vi "Main(Analysis_Debug2_Mode).vi"() -> ()   [LabVIEW 2015]
uses:
  Sub VI/buffer_mode.ctl
  <vilib>/Analysis/baseanly.llb/Mean (DBL).vi
  <vilib>/Utility/NIReport.llb/Append Text Table to Report (wrap).vi
  <vilib>/Utility/NIReport.llb/NI_report.lvclass
  <vilib>/Analysis/NI_AALBase.lvlib
panel:
  in  "Data Range Clear":bool
  in  "Auto Range":bool
  out "Range(min)":dbl caption="End - Start Time (min)"
  in  "Cursor Mode":enum16{"Free", "Sample"}(ring)
  out "Save as Task Time(sec)":dbl
  in  "Use Filter data":bool
  in  "Data Range Subset":bool
  in  "Range":dbl caption="Sample Range"
  in  "Analysis List":i32(listbox)
  in  "Data Range Addition":bool
  in  "Over-write":bool
  in  "Number of Data Down-Sampling":i32
  in  "Save As":bool
  in  "Refresh":bool
  in  "Delete":bool
  in  "Plot Display mode":T1(ring)
  in  "File Name":string(combo)
  in  "Analysis mode":u16(ring) items=["Sensor Response Linearity", "Sensor Hysteresis with No Dwell Time", "Sensor Hysteresis with Varying Dwell Time", "Reated Loading", "Drift with Set Temperature and Voltage", "Variation Due to Self-Heating", "Variation with Changing Voltage", "Electrical Noise"]
  in  "Start Analysis":bool
  in  "File Path":path
  out "XY 그래프":cluster{"Time(s)":dbl[], "calculation":u32[]}[](graph)
  # "V1.0"
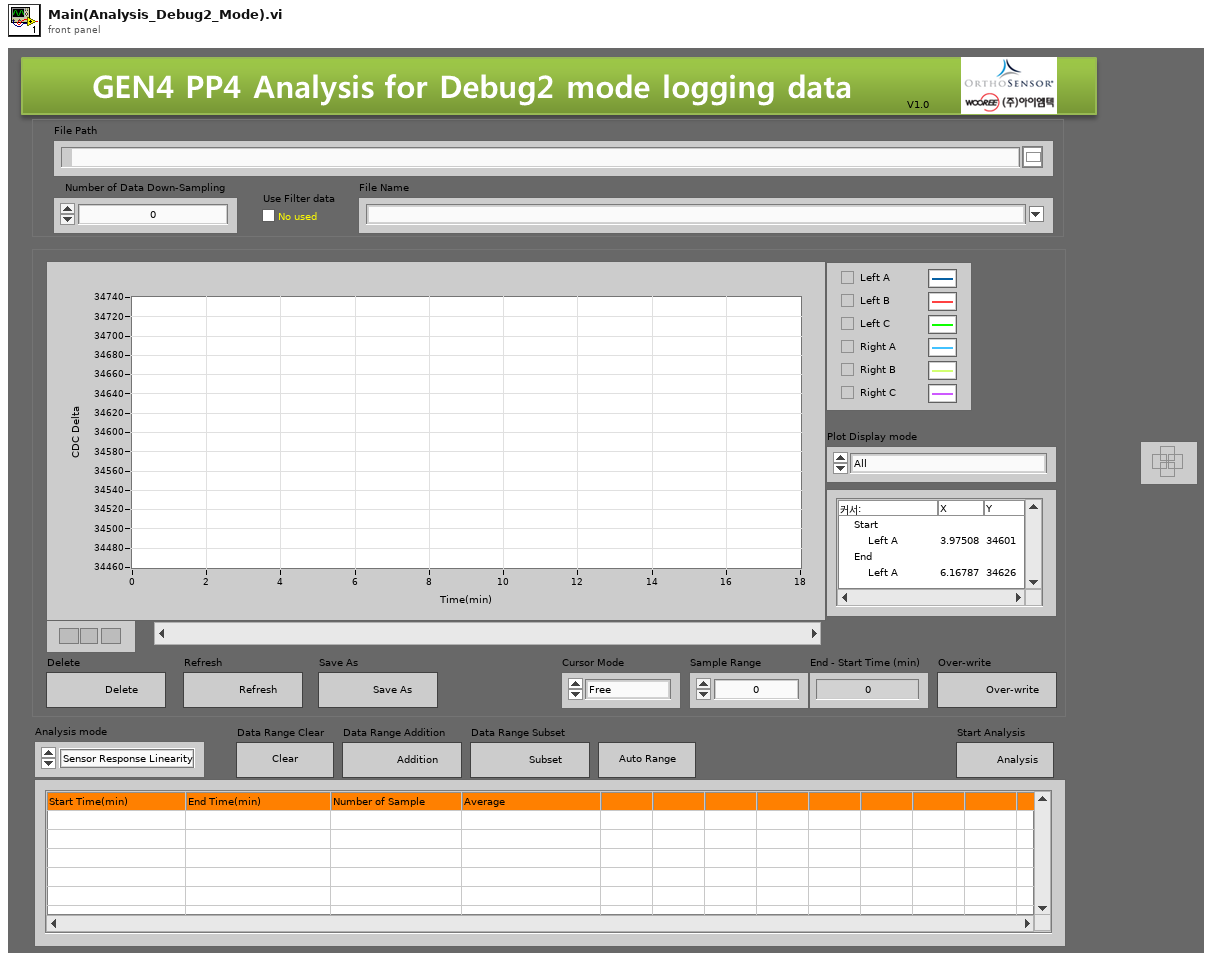
[diagram p1: front panel]
types:
  T1 = enum16{"All", "Left A", "Left B", "Left C", "Right A", "Right B", "Right C"}
  T2 = enum8{"Enabled", "Disabled", "Disabled and Grayed Out"}
  T3 = typedef "LVCursorListTypeDef.ctl" = cluster{"Name":string, "Color":u32, "Style":u8, "Point Style":u8, "Name Visible":bool, "Allow Drag":bool, "Cursor Mode":u32, "Plot":i32, "Index":i32, "Position":cluster{"X":dbl, "Y":dbl}, "X Scale":u32, "Y Scale":u32, "Watch Plots":i32[], "Watch All Plots":bool, "Plot Area":i32, "Label Offset":cluster{"X":dbl, "Y":dbl}}[]
  T4 = cluster{"Name":string, "Color":u32, "Style":u8, "Point Style":u8, "Name Visible":bool, "Allow Drag":bool, "Cursor Mode":u32, "Plot":i32, "Index":i32, "Position":cluster{"X":dbl, "Y":dbl}, "X Scale":u32, "Y Scale":u32, "Watch Plots":i32[], "Watch All Plots":bool, "Plot Area":i32, "Label Offset":cluster{"X":dbl, "Y":dbl}}
  T5 = typedef "buffer_mode.ctl" = enum16{"Clear", "Init", "Add 2nd data", "Delete", "Output"}
  T6 = cluster{"position (excel)":cluster{"row":i32, "column":i32}, "name (excel)":string, "bookmark (word)":string}
  T7 = enum16{"maximized", "minimized", "normal", "no change"}
  T8 = enum16{"Standard Report", "HTML", "Word", "Excel"}
  T9 = cluster{"Name":string, "Color":u32, "Style":u8, "Point Style":u8, "Name Visible":bool, "Allow Drag":bool, "Cursor Mode":u32, "Plot":i32, "Index":i32, "Position":cluster{"X":dbl, "Y":dbl}, "X Scale":u32, "Y Scale":u32, "Watch Plots":i32[], "Watch All Plots":bool, "Plot Area":i32, "Label Offset":cluster{"X":dbl, "Y":dbl}}[]
  T10 = cluster{"Timeline out":dbl[], "Counts out":u32[]}
  T11 = cluster{"Timeline out":dbl[], "Counts out":u32[]}[]
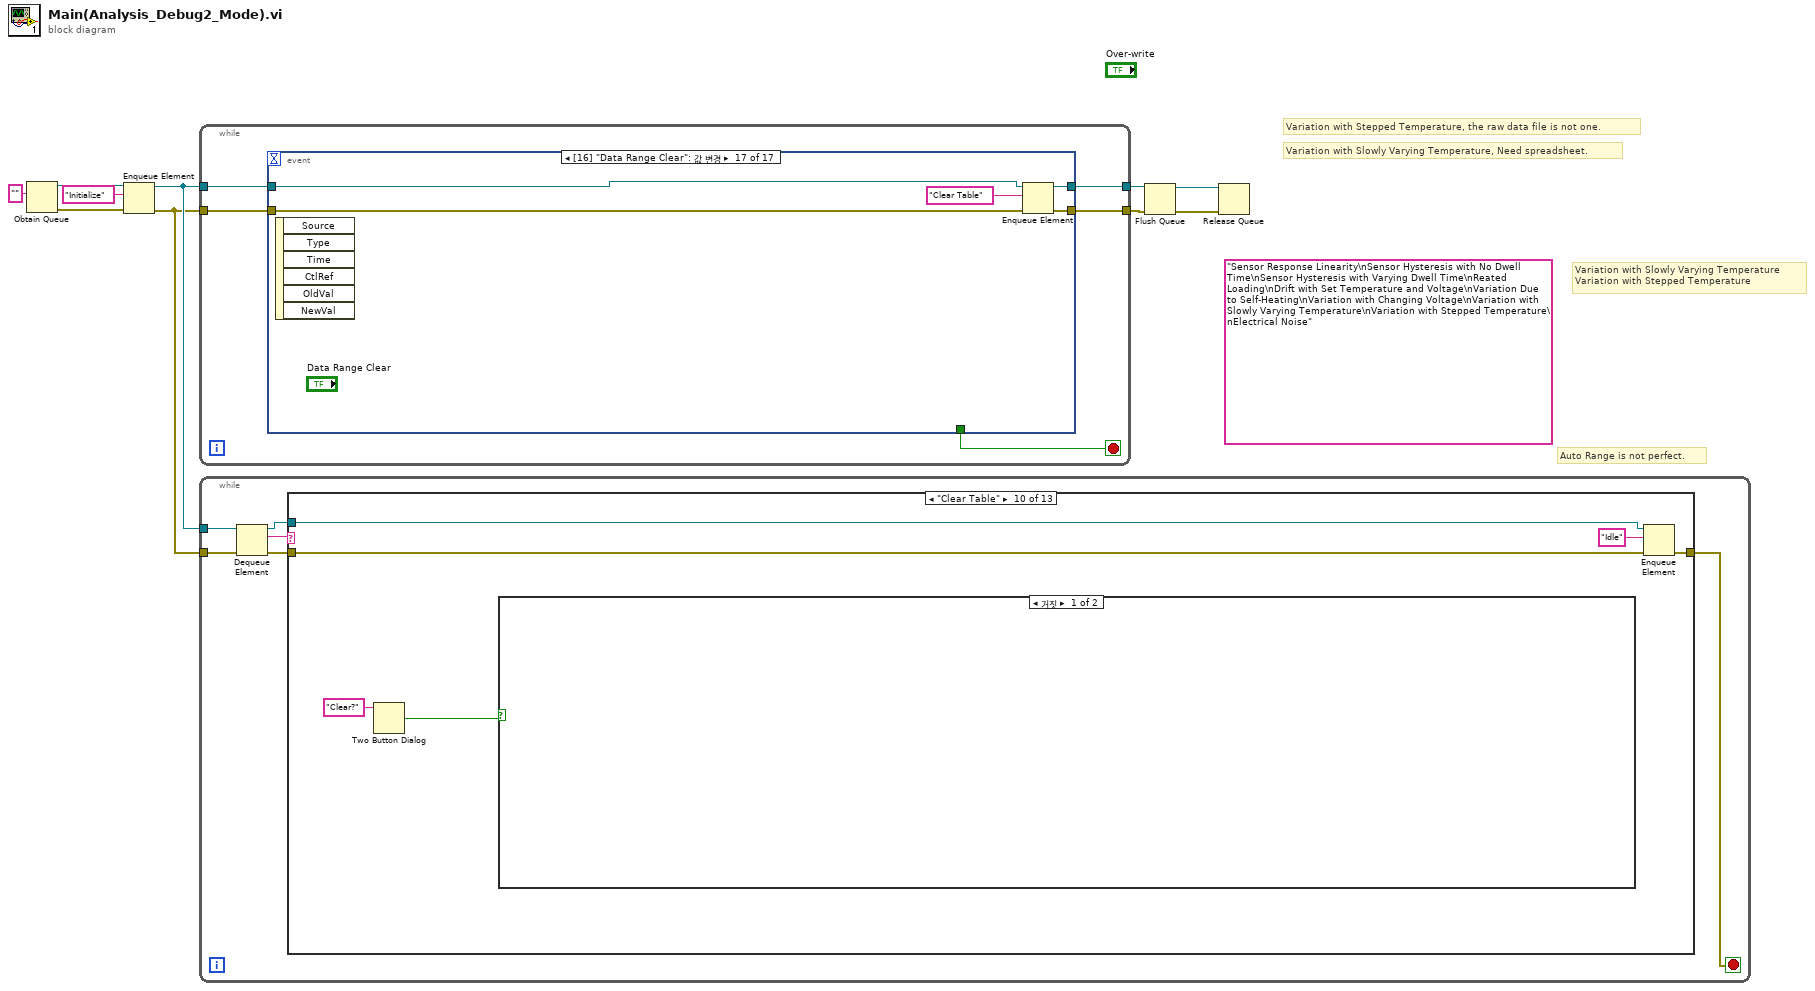
[diagram p0: block diagram]
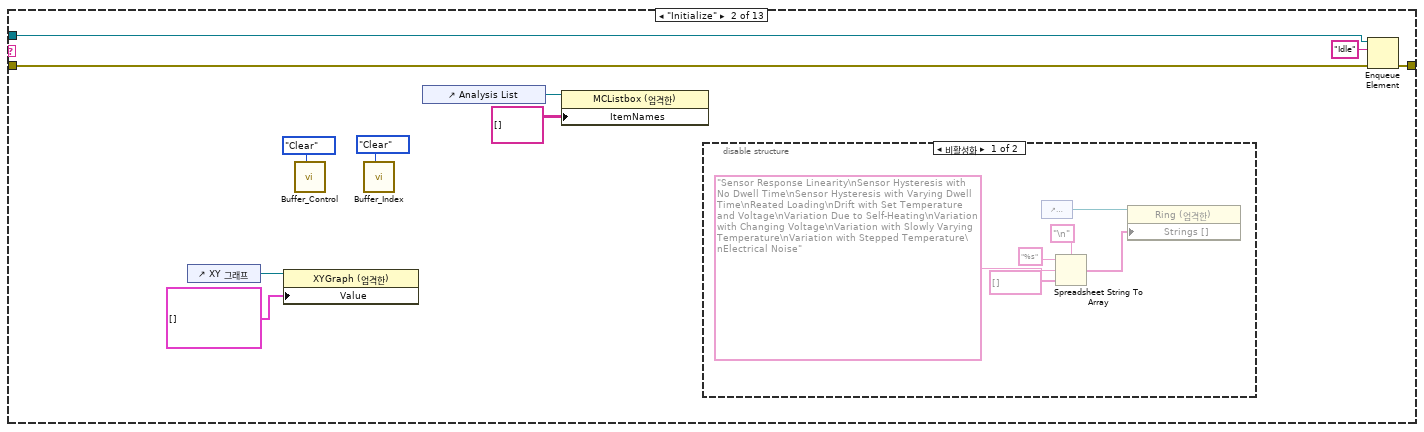
[diagram p3: hidden frame]
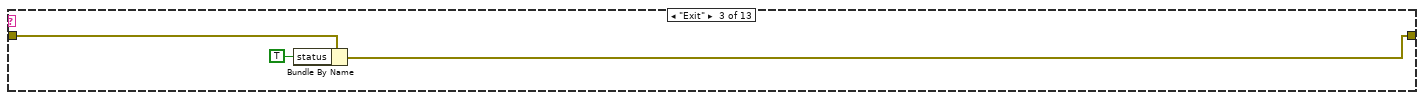
[diagram p5: hidden frame]
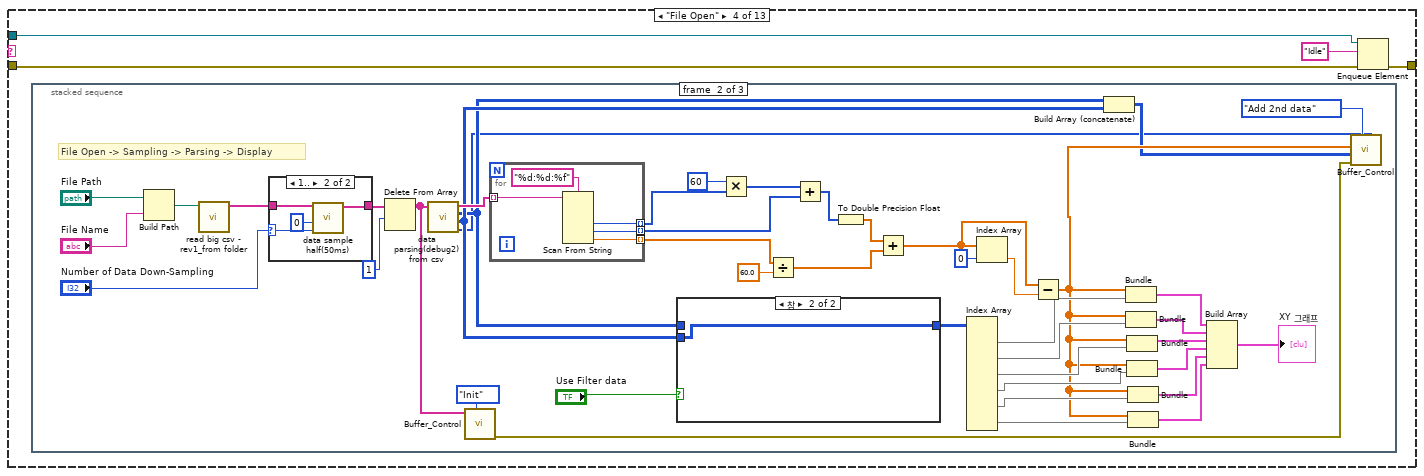
[diagram p6: hidden frame]
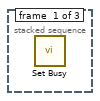
[diagram p7: hidden frame]
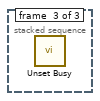
[diagram p10: hidden frame]
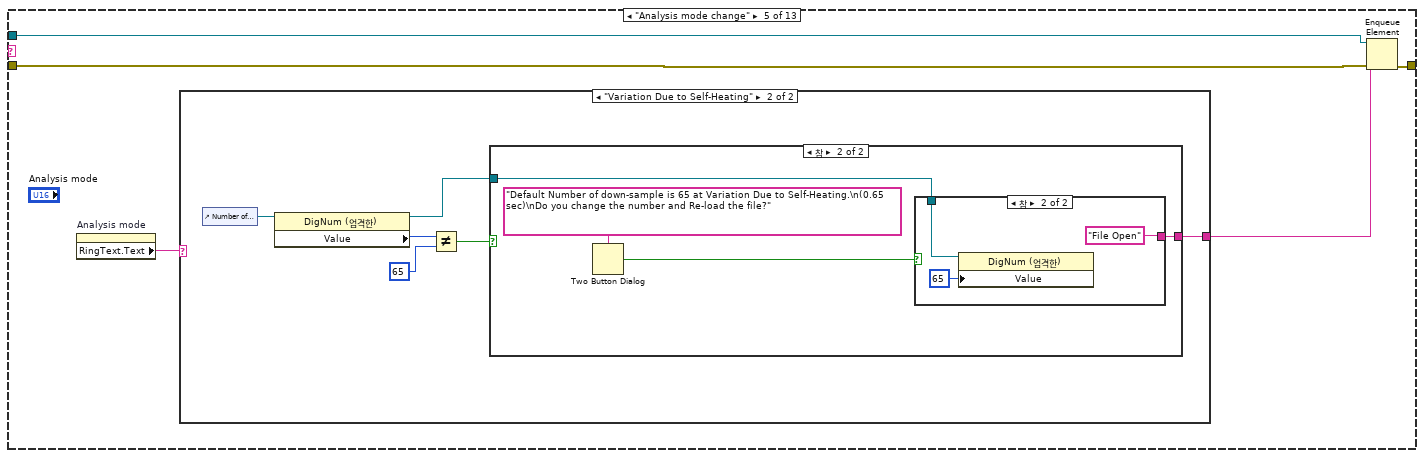
[diagram p11: hidden frame]
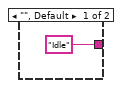
[diagram p12: hidden frame]
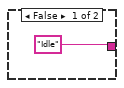
[diagram p13: hidden frame]
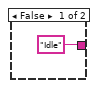
[diagram p14: hidden frame]
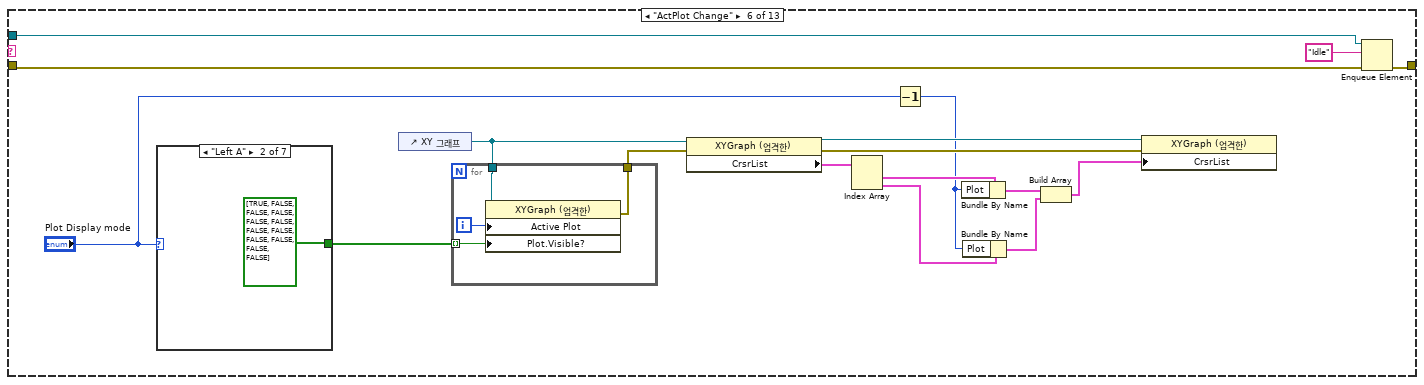
[diagram p15: hidden frame]
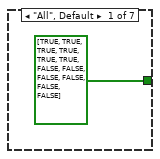
[diagram p16: hidden frame]
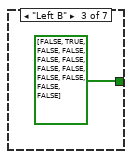
[diagram p17: hidden frame]
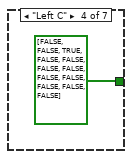
[diagram p18: hidden frame]
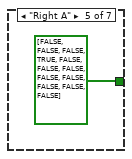
[diagram p19: hidden frame]
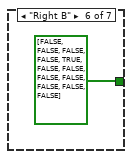
[diagram p20: hidden frame]
diagram:
  (unwired) "Sensor Response Linearity\nSensor Hysteresis with No Dwell Time\nSensor Hysteresis with Varying Dwell Time\nReated Loading\nDrift with Set Temperature and Voltage\nVariation Due to Self-Heating\nVariation with Changing Voltage\nVariation with Slowly Varying Temperature\nVariation with Stepped Temperature\nElectrical Noise" ("스프레드시트 문자열")
  # "Variation with Slowly Varying Temperature, Need spreadsheet."
  # "Variation with Stepped Temperature, the raw data file is not one."
  # "Variation with Slowly Varying Temperature\nVariation with Stepped Temperature"
  # "Auto Range is not perfect."
  n1 = Obtain Queue(element data type="" ("element")) -> (queue out=w10:refnum<queue>, error out=w9:errorcluster)  [unwired: 4 in, 1 out]
  n2 = Enqueue Element(queue=w10, element="Initialize", error in (no error)=w9) -> (queue out=w2:refnum<queue>, error out=w1:errorcluster)  [unwired: 1 in, 1 out]
  n3 = while {
    tunnel: w2 -> [w15]
    tunnel: [w14] -> w4
    tunnel: w1 -> [w13]
    tunnel: [w12] -> w3
    stop <- w11 stop-if-true
    n4 = event shown="[16] \"Data Range Clear\": 값 변경" {
      selector: _ -> [_ _ _ _ _ _ _ _ _ _ _ _ _ _ _ _ _]
      dyn-events: _ -> [_ _ _ _ _ _ _ _ _ _ _ _ _ _ _ _ _]
      timeout: _ -> [_ _ _ _ _ _ _ _ _ _ _ _ _ _ _ _ _]
      tunnel: w15 -> [w17 w18 w26 w31 w39 w51 w67 w72 w77 w85 w94 w98 w108 w112 w119 w124 w130]
      tunnel: [w17 w20 w28 w33 w38 w52 w68 w73 w78 w88 w95 w101 w109 w114 w122 w126 w131] -> w14
      tunnel: w13 -> [w16 w19 w27 w32 w40 w50 w66 w71 w76 w86 w93 w99 w107 w113 w120 w125 w129]
      tunnel: [w16 w21 w29 w34 w41 w53 w69 w74 w79 w87 w96 w100 w110 w115 w121 w127 w132] -> w12
      tunnel: [_ TRUE _ _ _ _ _ _ _ _ _ _ _ _ _ _ _] -> w11
      event Timeout {
        n5 = event-data() -> ()  [unwired: 1 in, 3 out]
      }
      event Panel Close {
        n6 = event-data() -> ()  [unwired: 1 in, 4 out]
        n7 = Enqueue Element(queue=w18, element="Exit", error in (no error)=w19) -> (queue out=w20:refnum<queue>, error out=w21:errorcluster)  [unwired: 1 in, 1 out]
      }
      event "File Name": Value Change {
        # "File Open -> Sampling -> Parsing -> Display"
        n8 = event-data() -> ()  [unwired: 1 in, 1 out]
        n9 = control-ref of="XY 그래프"() -> (w25:refnum<vi>)
        n10 = property class="XYGraph (엄격한)"(reference=w25, "Value"=cluster{"Time(s)":dbl[], "calculation":u32[]}[] [] ("값")) -> ()  [unwired: 1 in, 2 out]
        n11 = Enqueue Element(queue=w26, element="File Open", error in (no error)=w27) -> (queue out=w28:refnum<queue>, error out=w29:errorcluster)  [unwired: 1 in, 1 out]
      }
      event "Delete": Value Change {
        n12 = event-data() -> ()  [unwired: 1 in, 6 out]
        n13 = Enqueue Element(queue=w31, element="Delete DATA", error in (no error)=w32) -> (queue out=w33:refnum<queue>, error out=w34:errorcluster)  [unwired: 1 in, 1 out]
      }
      event "Cursor Mode": Value Change {
        n14 = event-data() -> ()  [unwired: 1 in, 6 out]
        n15 = local read "Cursor Mode"() -> (w36:enum16{"Free", "Sample"})
        n16 = control-ref of="Range"() -> (w37:refnum<vi>)
        n17 = case shown="\"Free\", 기본" w36 {
          tunnel: w37 -> [w44 w47]
          frame "Free", Default {
            n18 = property class="DigNum (엄격한)"(reference=w44, "DisabledEnum"=T2."Disabled and Grayed Out" ("비활성화")) -> ()  [unwired: 1 in, 2 out]
          }
          frame "Sample" {
            n19 = property class="DigNum (엄격한)"(reference=w47, "Caption.Text"="Sample Range" ("캡션.텍스트"), "DisabledEnum"=T2."Enabled" ("비활성화")) -> ()  [unwired: 1 in, 2 out]
          }
        }
        n20 = Enqueue Element(queue=w39, element="Idle", error in (no error)=w40) -> (queue out=w38:refnum<queue>, error out=w41:errorcluster)  [unwired: 1 in, 1 out]
      }
      event "XY 그래프": Cursor Move {
        n21 = event-data() -> ("CursRef"=w49:refnum<vi>)  [unwired: 1 in, 8 out]
        n22 = flat-sequence {
          tunnel: w49 -> [w58]
          tunnel: [w55] -> w48
          tunnel: w48 -> [w59]
          frame #0 {
            n23 = control-ref of="XY 그래프"() -> (w55:refnum<vi>)
            n24 = call "Sub_Cursor_Control.vi"("Range"="Range", "XY 그래프"=w55, "CursRef"=w58, "Cursor Mode"="Cursor Mode") -> ()  [unwired: 8 in]
          }
          frame #1 {
            n25 = property class="XYGraph (엄격한)"(reference=w59) -> ("CrsrList"=w65:T3)  [unwired: 1 in, 2 out]
            n26 = Index Array(array=w65) -> (element #1=w64:T4, element #2=w63:T4)  [unwired: 2 in]
            n27 = Unbundle By Name(w64) -> ("Position.X"=w62:dbl)
            n28 = Unbundle By Name(w63) -> ("Position.X"=w61:dbl)
            n29 = Subtract(x=w61, y=w62) -> (x-y=→"Range(min)":dbl)
          }
        }
        n30 = Enqueue Element(queue=w51, element="Idle", error in (no error)=w50) -> (queue out=w52:refnum<queue>, error out=w53:errorcluster)  [unwired: 1 in, 1 out]
      }
      event "Data Range Addition": Value Change {
        n31 = event-data() -> ()  [unwired: 1 in, 6 out]
        n32 = Enqueue Element(queue=w67, element="Add data to Table", error in (no error)=w66) -> (queue out=w68:refnum<queue>, error out=w69:errorcluster)  [unwired: 1 in, 1 out]
      }
      event "Analysis List": Mouse Down {
        n33 = event-data() -> ()  [unwired: 1 in, 8 out]
        n34 = Enqueue Element(queue=w72, element="Move to Cursor", error in (no error)=w71) -> (queue out=w73:refnum<queue>, error out=w74:errorcluster)  [unwired: 1 in, 1 out]
      }
      event "Analysis mode": Value Change {
        n35 = event-data() -> ()  [unwired: 1 in, 6 out]
        n36 = Enqueue Element(queue=w77, element="Analysis mode change", error in (no error)=w76) -> (queue out=w78:refnum<queue>, error out=w79:errorcluster)  [unwired: 1 in, 1 out]
      }
      event "Data Range Subset": Value Change {
        n37 = event-data() -> ()  [unwired: 1 in, 6 out]
        n38 = control-ref of="Analysis List"() -> (w90:refnum<vi>)
        n39 = property class="MCListbox (엄격한)"(reference=w90) -> (reference out=w84:refnum<vi>, "FocusRow"=w81:i32, "ItemNames"=w91:string[][])  [unwired: 1 in, 1 out]
        n40 = call "Buffer_Index.vi"("Mode"=enum16{"Clear", "Add", "Del"}."Del", "Delete Position(row)"=w81) -> ()  [unwired: 9 in, 1 out]
        n41 = Delete From Array(array=w91, length=1 ("길이"), index (row)=w81) -> (array with subset deleted=w83:string[][])  [unwired: 1 in, 1 out]
        n42 = property class="MCListbox (엄격한)"(reference=w84, "ItemNames"=w83) -> ()  [unwired: 1 in, 2 out]
        n43 = Enqueue Element(queue=w85, element="Idle", error in (no error)=w86) -> (queue out=w88:refnum<queue>, error out=w87:errorcluster)  [unwired: 1 in, 1 out]
      }
      event "Auto Range": Value Change {
        n44 = event-data() -> ()  [unwired: 1 in, 6 out]
        n45 = Enqueue Element(queue=w94, element="Auto Range Setting", error in (no error)=w93) -> (queue out=w95:refnum<queue>, error out=w96:errorcluster)  [unwired: 1 in, 1 out]
      }
      event "File Path": Value Change {
        n46 = event-data() -> ("NewVal"=w106:path)  [unwired: 1 in]
        n47 = List Folder(path=w106, pattern="*.csv" ("패턴")) -> (filenames=w104:string[])  [unwired: 2 in, 3 out]
        n48 = control-ref of="File Name"() -> (w105:refnum<vi>)
        n49 = property class="CmbBox"(reference=w105, "Strings[]"=w104) -> ()  [unwired: 1 in, 2 out]
        n50 = Enqueue Element(queue=w98, element="Idle", error in (no error)=w99) -> (queue out=w101:refnum<queue>, error out=w100:errorcluster)  [unwired: 1 in, 1 out]
      }
      event "Plot Display mode": Value Change {
        n51 = event-data() -> ()  [unwired: 1 in, 6 out]
        n52 = Enqueue Element(queue=w108, element="ActPlot Change", error in (no error)=w107) -> (queue out=w109:refnum<queue>, error out=w110:errorcluster)  [unwired: 1 in, 1 out]
      }
      event "Refresh": Value Change {
        n53 = event-data() -> ()  [unwired: 1 in, 6 out]
        n54 = control-ref of="XY 그래프"() -> (w118:refnum<vi>)
        n55 = property class="XYGraph (엄격한)"(reference=w118, "ActPaletteTool"=5 ("팔레트:활성 도구")) -> ()  [unwired: 1 in, 2 out]
        n56 = Enqueue Element(queue=w112, element="Idle", error in (no error)=w113) -> (queue out=w114:refnum<queue>, error out=w115:errorcluster)  [unwired: 1 in, 1 out]
      }
      event "Save As": Value Change {
        n57 = event-data() -> ()  [unwired: 1 in, 1 out]
        n58 = Enqueue Element(queue=w119, element="Save as", error in (no error)=w120) -> (queue out=w122:refnum<queue>, error out=w121:errorcluster)  [unwired: 1 in, 1 out]
      }
      event "Start Analysis": Value Change {
        n59 = event-data() -> ()  [unwired: 1 in, 6 out]
        n60 = Enqueue Element(queue=w124, element="Analysis", error in (no error)=w125) -> (queue out=w126:refnum<queue>, error out=w127:errorcluster)  [unwired: 1 in, 1 out]
      }
      event "Data Range Clear": Value Change {
        n61 = event-data() -> ()  [unwired: 1 in, 6 out]
        n62 = Enqueue Element(queue=w130, element="Clear Table", error in (no error)=w129) -> (queue out=w131:refnum<queue>, error out=w132:errorcluster)  [unwired: 1 in, 1 out]
      }
    }
  }
  n63 = while {
    tunnel: w2 -> [w138]
    tunnel: w1 -> [w137]
    stop <- w134 stop-if-true
    n64 = Dequeue Element(queue=w138, error in (no error)=w137) -> (queue out=w135:refnum<queue>, element=w139:string, error out=w136:errorcluster)  [unwired: 1 in, 1 out]
    n65 = case shown="\"Clear Table\"" w139 {
      tunnel: w136 -> [w140 w149 w159 w162 w222 w255 w272 w286 w335 w398 w406 w551 w570]
      tunnel: w135 -> [_ w148 _ w161 w223 w254 w271 w285 w334 w397 w405 w550 w569]
      tunnel: [w140 w147 w157 w163 w224 w256 w273 w287 w336 w399 w407 w552 w571] -> w134
      frame "Idle", Default {
      }
      frame "Initialize" {
        n66 = control-ref of="XY 그래프"() -> (w145:refnum<vi>)
        n67 = property class="XYGraph (엄격한)"(reference=w145, "Value"=cluster{"Time(s)":dbl[], "calculation":u32[]}[] [] ("값")) -> ()  [unwired: 1 in, 2 out]
        n68 = call "Buffer_Control.vi"("Mode"=buffer_mode."Clear") -> ()  [unwired: 6 in, 5 out]
        n69 = call "Buffer_Index.vi"("Mode"=enum16{"Clear", "Add", "Del"}."Clear") -> ()  [unwired: 10 in, 1 out]
        n70 = control-ref of="Analysis List"() -> (w142:refnum<vi>)
        n71 = property class="MCListbox (엄격한)"(reference=w142, "ItemNames"=string[][] []) -> ()  [unwired: 1 in, 2 out]
        n72 = disable-structure shown="비활성화" {
          frame Disabled {
            n73 = control-ref of="Analysis mode"() -> (w156:refnum<vi>)
            n74 = Spreadsheet String To Array(delimiter (Tab)="\n" ("구분 문자(탭)"), format string="%s" ("포맷 문자열"), spreadsheet string="Sensor Response Linearity\nSensor Hysteresis with No Dwell Time\nSensor Hysteresis with Varying Dwell Time\nReated Loading\nDrift with Set Temperature and Voltage\nVariation Due to Self-Heating\nVariation with Changing Voltage\nVariation with Slowly Varying Temperature\nVariation with Stepped Temperature\nElectrical Noise" ("스프레드시트 문자열"), array type (2D Dbl)=string[] []) -> (array=w152:string[])
            n75 = property class="Ring (엄격한)"(reference=w156, "Strings []"=w152) -> ()  [unwired: 1 in, 2 out]
          }
          frame Enabled {
          }
        }
        n76 = Enqueue Element(queue=w148, element="Idle", error in (no error)=w149) -> (error out=w147:errorcluster)  [unwired: 1 in, 2 out]
      }
      frame "Exit" {
        n77 = Bundle By Name(cluster=w159, "status"=TRUE) -> (w157:errorcluster)
      }
      frame "File Open" {
        n78 = stacked-sequence {
          frame #0 {
            n79 = call <vilib>:"Set Busy.vi"() -> ()  [unwired: 10 in, 2 out]
          }
          frame #1 {
            # "File Open -> Sampling -> Parsing -> Display"
            n80 = Build Path(base path="File Path", name or relative path="File Name") -> (appended path=w205:path)
            n81 = call "read big csv - rev1_from folder.vi"("파일 경로(대화 상자 사용)"=w205) -> ("배열"=w204:string[])  [unwired: 10 in]
            n82 = case shown="1.." "Number of Data Down-Sampling" {
              selector: "Number of Data Down-Sampling" -> [_ w218]
              tunnel: w204 -> [w215 w219]
              tunnel: [w215 w217] -> w175
              frame 0, Default {
              }
              frame 1.. {
                n83 = call "data sample half(50ms).vi"("Number of Remove data"=w218, "Offset"=0, "Array"=w219) -> ("Array out"=w217:string[])  [unwired: 8 in]
              }
            }
            n84 = Delete From Array(array=w175, length=1 ("길이")) -> (array with subset deleted=w171:string[])  [unwired: 1 in, 1 out]
            n85 = call "data parsing(debug2) from csv.vi"("배열"=w171) -> ("Temp"=w164:u32[], "Filtered Sensor"=w167:u32[][], "No Filter Sensor"=w166:u32[][], "Time"=w173:string[])  [unwired: 7 in]
            n86 = call "Buffer_Control.vi"("Mode"=buffer_mode."Init", "Init input"=w171) -> ("error out"=w170:errorcluster)  [unwired: 5 in, 4 out]
            n87 = for {
              tunnel: w173 -> [w214] mode=indexing
              tunnel: [w212] -> w191 mode=indexing
              tunnel: [w211] -> w196 mode=indexing
              tunnel: [w210] -> w195 mode=indexing
              n88 = Scan From String(format string="%d:%d:%f" ("포맷 문자열"), input string=w214) -> (output 1=w212:i32, output 2=w211:i32, output 3=w210:dbl)  [unwired: 5 in, 3 out]
            }
            n89 = case shown="참" "Use Filter data" {
              tunnel: w166 -> [w208 _]
              tunnel: w167 -> [_ w209]
              tunnel: [w208 w209] -> w189
              frame False {
              }
              frame True {
              }
            }
            n90 = Multiply(x=60, y=w191) -> (x*y=w202:i32[])
            n91 = Divide(x=w195, y=60.0) -> (x/y=w193:dbl[])
            n92 = Add(x=w202, y=w196) -> (x+y=w200:i32[])
            n93 = To Double Precision Float(number=w200) -> (double precision float=w201:dbl[])
            n94 = Add(x=w201, y=w193) -> (x+y=w197:dbl[])
            n95 = Index Array(array=w189) -> (element #1=w188:u32[], element #2=w187:u32[], element #3=w186:u32[], element #4=w185:u32[], element #5=w184:u32[], element #6=w183:u32[])  [unwired: 12 in]
            n96 = Index Array(array=w197, index=0 ("인덱스")) -> (element=w198:dbl)
            n97 = Subtract(x=w197, y=w198) -> (x-y=w169:dbl[])
            n98 = Build Array (concatenate)(w166, w167) -> (w165:u32[][])
            n99 = Bundle(w169, "Filtered Sensor"=w188) -> (w182:cluster{dbl[], "Filtered Sensor":u32[]})  [unwired: 1 in]
            n100 = Bundle(w169, "Filtered Sensor"=w187) -> (w181:cluster{dbl[], "Filtered Sensor":u32[]})  [unwired: 1 in]
            n101 = Bundle(w169, "Filtered Sensor"=w186) -> (w180:cluster{dbl[], "Filtered Sensor":u32[]})  [unwired: 1 in]
            n102 = Bundle(w169, "Filtered Sensor"=w185) -> (w179:cluster{dbl[], "Filtered Sensor":u32[]})  [unwired: 1 in]
            n103 = Bundle(w169, "Filtered Sensor"=w184) -> (w178:cluster{dbl[], "Filtered Sensor":u32[]})  [unwired: 1 in]
            n104 = Bundle(w169, "Filtered Sensor"=w183) -> (w177:cluster{dbl[], "Filtered Sensor":u32[]})  [unwired: 1 in]
            n105 = Build Array(w182, w181, w180, w179, w178, w177) -> (→"XY 그래프":cluster{dbl[], "Filtered Sensor":u32[]}[])
            n106 = call "Buffer_Control.vi"("Temp"=w164, "Mode"=buffer_mode."Add 2nd data", "error in (no error)"=w170, "Counts"=w165, "Timeline"=w169) -> ()  [unwired: 2 in, 5 out]
          }
          frame #2 {
            n107 = call <vilib>:"Unset Busy.vi"() -> ()  [unwired: 11 in, 1 out]
          }
        }
        n108 = Enqueue Element(queue=w161, element="Idle", error in (no error)=w162) -> (error out=w163:errorcluster)  [unwired: 1 in, 2 out]
      }
      frame "Analysis mode change" {
        n109 = property on="Analysis mode" class="Ring (엄격한)"() -> ("RingText.Text"=w221:string)  [unwired: 2 in, 2 out]
        n110 = case shown="\"Variation Due to Self-Heating\"" w221 {
          tunnel: ["Idle" ("element") w226] -> w220
          frame "", Default {
          }
          frame "Variation Due to Self-Heating" {
            n111 = control-ref of="Number of Data Down-Sampling"() -> (w231:refnum<vi>)
            n112 = property class="DigNum (엄격한)"(reference=w231) -> (reference out=w227:refnum<vi>, "Value"=w230:i32)  [unwired: 1 in, 1 out]
            n113 = Not Equal?(x=w230, y=65) -> (x != y?=w228:bool)
            n114 = case shown="참" w228 {
              tunnel: w227 -> [_ w235]
              tunnel: ["Idle" w233] -> w226
              frame False {
              }
              frame True {
                n115 = Two Button Dialog(message="Default Number of down-sample is 65 at Variation Due to Self-Heating.\n(0.65 sec)\nDo you change the number and Re-load the file?" ("메시지")) -> (T button?=w234:bool)  [unwired: 2 in]
                n116 = case shown="참" w234 {
                  tunnel: w235 -> [_ w240]
                  tunnel: ["Idle" ("element") "File Open"] -> w233
                  frame False {
                  }
                  frame True {
                    n117 = property class="DigNum (엄격한)"(reference=w240, "Value"=65 ("값")) -> ()  [unwired: 1 in, 2 out]
                  }
                }
              }
            }
          }
        }
        n118 = Enqueue Element(queue=w223, element=w220, error in (no error)=w222) -> (error out=w224:errorcluster)  [unwired: 1 in, 2 out]
      }
      frame "ActPlot Change" {
        n119 = case shown="\"Left A\"" "Plot Display mode" {
          tunnel: [bool[] [TRUE, TRUE, TRUE, TRUE, TRUE, TRUE, FALSE, FALSE, FALSE, FALSE, FALSE, FALSE] ("Select") bool[] [TRUE, FALSE, FALSE, FALSE, FALSE, FALSE, FALSE, FALSE, FALSE, FALSE, FALSE, FALSE] ("Select") bool[] [FALSE, TRUE, FALSE, FALSE, FALSE, FALSE, FALSE, FALSE, FALSE, FALSE, FALSE, FALSE] ("Select") bool[] [FALSE, FALSE, TRUE, FALSE, FALSE, FALSE, FALSE, FALSE, FALSE, FALSE, FALSE, FALSE] ("Select") bool[] [FALSE, FALSE, FALSE, TRUE, FALSE, FALSE, FALSE, FALSE, FALSE, FALSE, FALSE, FALSE] ("Select") bool[] [FALSE, FALSE, FALSE, FALSE, TRUE, FALSE, FALSE, FALSE, FALSE, FALSE, FALSE, FALSE] ("Select") bool[] [FALSE, FALSE, FALSE, FALSE, FALSE, TRUE, FALSE, FALSE, FALSE, FALSE, FALSE, FALSE] ("Select")] -> w253
          frame "All", Default {
          }
          frame "Left A" {
          }
          frame "Left B" {
          }
          frame "Left C" {
          }
          frame "Right A" {
          }
          frame "Right B" {
          }
          frame "Right C" {
          }
        }
        n120 = control-ref of="XY 그래프"() -> (w252:refnum<vi>)
        n121 = for {
          tunnel: w252 -> [w261]
          tunnel: w253 -> [w259] mode=indexing
          tunnel: [w258] -> w248
          i -> [w260]
          n122 = property class="XYGraph (엄격한)"(reference=w261, "Active Plot"=w260, "Plot.Visible?"=w259) -> (error out=w258:errorcluster)  [unwired: 1 in, 1 out]
        }
        n123 = property class="XYGraph (엄격한)"(reference=w252, error in=w248) -> (reference out=w243:refnum<vi>, error out=w242:errorcluster, "CrsrList"=w251:T3)
        n124 = Index Array(array=w251) -> (element #1=w250:T4, element #2=w249:T4)  [unwired: 2 in]
        n125 = Decrement(x="Plot Display mode") -> (x-1=w241:T1)
        n126 = Bundle By Name(cluster=w250, "Plot"=w241) -> (w246:T4)
        n127 = Bundle By Name(cluster=w249, "Plot"=w241) -> (w245:T4)
        n128 = Build Array(w246, w245) -> (w244:T9)
        n129 = property class="XYGraph (엄격한)"(reference=w243, error in=w242, "CrsrList"=w244) -> ()  [unwired: 2 out]
        n130 = Enqueue Element(queue=w254, element="Idle", error in (no error)=w255) -> (error out=w256:errorcluster)  [unwired: 1 in, 2 out]
      }
      frame "Save as" {
        n131 = flat-sequence {
          tunnel: [w275] -> w270
          tunnel: w270 -> [w278]
          tunnel: [w278] -> w269
          tunnel: w269 -> [w283]
          frame #0 {
            n132 = Get Date/Time In Seconds() -> (seconds since 1Jan1904=w275:timestamp)
            n133 = call <vilib>:"Set Busy.vi"() -> ()  [unwired: 10 in, 2 out]
          }
          frame #1 {
            n134 = control-ref of="File Name"() -> (w279:refnum<vi>)
            n135 = control-ref of="File Path"() -> (w280:refnum<vi>)
            n136 = call "Sub_Saveas.vi"("Template Name"="saveas.xlsx" ("이름 또는 상대 경로"), "row"=2, "File Name"=w279, "Path"=w280) -> ()  [unwired: 7 in, 1 out]
          }
          frame #2 {
            n137 = Get Date/Time In Seconds() -> (seconds since 1Jan1904=w282:timestamp)
            n138 = Subtract(x=w282, y=w283) -> (x-y=→"Save as Task Time(sec)":dbl)
          }
          frame #3 {
            n139 = call <vilib>:"Unset Busy.vi"() -> ()  [unwired: 11 in, 1 out]
            n140 = One Button Dialog(message="Done~!!" ("메시지")) -> ()  [unwired: 1 in, 1 out]
          }
        }
        n141 = Enqueue Element(queue=w271, element="Idle", error in (no error)=w272) -> (error out=w273:errorcluster)  [unwired: 1 in, 2 out]
      }
      frame "Delete DATA" {
        n142 = stacked-sequence {
          seq-local: [w292 _] -> [_ w299]
          seq-local: [w290 _] -> [_ w298]
          seq-local: [w289 _] -> [_ w297]
          frame #0 {
            # "Length = End Index - Start Index"
            n143 = control-ref of="XY 그래프"() -> (w296:refnum<vi>)
            n144 = property class="XYGraph (엄격한)"(reference=w296) -> ("CrsrList"=w295:T3)  [unwired: 1 in, 2 out]
            n145 = Index Array(array=w295) -> (element #1=w294:T4, element #2=w293:T4)  [unwired: 2 in]
            n146 = Unbundle By Name(w294) -> ("Index"=w289:i32)
            n147 = Unbundle By Name(w293) -> ("Index"=w291:i32)
            n148 = Subtract(x=w291, y=w289) -> (x-y=w290:i32)
            n149 = Greater Than 0?(x=w290) -> (x > 0?=w292:bool)
          }
          frame #1 {
            n150 = case shown="거짓" w299 {
              tunnel: w298 -> [_ w302]
              tunnel: w297 -> [_ w301]
              frame False {
                n151 = One Button Dialog(message="Start cursor x value must be less than End cursor." ("메시지")) -> ()  [unwired: 1 in, 1 out]
              }
              frame True {
                n152 = Bundle By Name(cluster=cluster{"Del_Length":i32, "Del_Position":i32} {"Del_Length"=0, "Del_Position"=0} ("Del"), "Del_Length"=w302, "Del_Position"=w301) -> (w304:cluster{"Del_Length":i32, "Del_Position":i32})
                n153 = call "Buffer_Control.vi"("Del"=w304, "Mode"=buffer_mode."Delete") -> ("error out"=w303:errorcluster)  [unwired: 5 in, 4 out]
                n154 = stacked-sequence {
                  tunnel: w303 -> [_ w330]
                  frame #0 {
                    n155 = control-ref of="XY 그래프"() -> (w308:refnum<vi>)
                    n156 = property class="XYGraph (엄격한)"(reference=w308, "Value"=cluster{"Time(s)":dbl[], "calculation":u32[]}[] [] ("값")) -> ()  [unwired: 1 in, 2 out]
                  }
                  frame #1 {
                    n157 = call "Buffer_Control.vi"("Mode"=buffer_mode."Output", "error in (no error)"=w330) -> ("Counts out"=w328:u32[][], "Timeline out"=w322:dbl[])  [unwired: 5 in, 3 out]
                    n158 = control-ref of="Use Filter data"() -> (w326:refnum<vi>)
                    n159 = property class="Bool (엄격한)"(reference=w326) -> ("Value"=w327:bool)  [unwired: 1 in, 2 out]
                    n160 = case shown="참" w327 {
                      tunnel: [0 ("인덱스 (행)") 6 ("인덱스 (행)")] -> w324
                      frame False {
                      }
                      frame True {
                      }
                    }
                    n161 = Delete From Array(array=w328, length=6 ("길이"), index (row)=w324) -> (deleted portion=w309:u32[][])  [unwired: 1 in, 1 out]
                    n162 = Index Array(array=w309) -> (element #1=w323:u32[], element #2=w321:u32[], element #3=w320:u32[], element #4=w319:u32[], element #5=w318:u32[], element #6=w317:u32[])  [unwired: 12 in]
                    n163 = Bundle("Timeline out"=w322, "Counts out"=w323) -> (w316:T10)  [unwired: 1 in]
                    n164 = Bundle("Timeline out"=w322, "Counts out"=w321) -> (w315:T10)  [unwired: 1 in]
                    n165 = Bundle("Timeline out"=w322, "Counts out"=w320) -> (w314:T10)  [unwired: 1 in]
                    n166 = Bundle("Timeline out"=w322, "Counts out"=w319) -> (w313:T10)  [unwired: 1 in]
                    n167 = Bundle("Timeline out"=w322, "Counts out"=w318) -> (w312:T10)  [unwired: 1 in]
                    n168 = Bundle("Timeline out"=w322, "Counts out"=w317) -> (w311:T10)  [unwired: 1 in]
                    n169 = Build Array(w316, w315, w314, w313, w312, w311) -> (w310:T11)
                    n170 = control-ref of="XY 그래프"() -> (w329:refnum<vi>)
                    n171 = property class="XYGraph (엄격한)"(reference=w329, "Value"=w310) -> ()  [unwired: 1 in, 2 out]
                  }
                }
              }
            }
          }
        }
        n172 = Enqueue Element(queue=w285, element="Idle", error in (no error)=w286) -> (error out=w287:errorcluster)  [unwired: 1 in, 2 out]
      }
      frame "Add data to Table" {
        n173 = stacked-sequence {
          seq-local: [w339 _ _] -> [_ _ w361]
          seq-local: [w340 _ _] -> [_ _ w362]
          seq-local: [w338 _ _] -> [_ _ w365]
          seq-local: [_ w348 _] -> [_ _ w363]
          seq-local: [_ w351 _] -> [_ _ w364]
          frame #0 {
            # "Detect empty line"
            n174 = control-ref of="Analysis List"() -> (w338:refnum<vi>)
            n175 = property class="MCListbox (엄격한)"(reference=w338) -> ("ItemNames"=w340:string[][])  [unwired: 1 in, 2 out]
            n176 = for {
              tunnel: w340 -> [w345] mode=indexing
              tunnel: [w341] -> w339
              i -> [w341]
              stop <- w342 stop-if-true
              # "Start Time = \"\""
              n177 = Index Array(array=w345) -> (element=w344:string)  [unwired: 1 in]
              n178 = Equal?(x=w344, y="") -> (x = y?=w342:bool)
            }
          }
          frame #1 {
            # "Search data will be used"
            n179 = control-ref of="Plot Display mode"() -> (w352:refnum<vi>)
            n180 = property class="Enum (엄격한)"(reference=w352) -> ("Value"=w346:T1)  [unwired: 1 in, 2 out]
            n181 = control-ref of="Use Filter data"() -> (w350:refnum<vi>)
            n182 = property class="Bool (엄격한)"(reference=w350) -> ("Value"=w349:bool)  [unwired: 1 in, 2 out]
            n183 = To Long Integer(number=w346) -> (32bit integer=w347:i32)
            n184 = case shown="\"Left A\", 기본" w346 {
              tunnel: [FALSE TRUE] -> w351
              frame "All" {
                n185 = One Button Dialog(message="Plot Display mode must be not All~!" ("메시지")) -> ()  [unwired: 1 in, 1 out]
              }
              frame "Left A", Default {
              }
            }
            n186 = case shown="거짓" w349 {
              tunnel: w347 -> [w354 w355]
              tunnel: [w353 w356] -> w348
              frame False {
                n187 = Decrement(x=w354) -> (x-1=w353:i32)
              }
              frame True {
                # "If Left A, 6\n1 + 5 = 6"
                n188 = Add(x=5, y=w355) -> (x+y=w356:i32)
              }
            }
          }
          frame #2 {
            # "Add data to Table"
            n189 = case shown="참" w364 {
              tunnel: w365 -> [_ w388]
              tunnel: w363 -> [_ w386]
              tunnel: w362 -> [_ w374]
              tunnel: w361 -> [_ w373]
              frame False {
              }
              frame True {
                n190 = control-ref of="XY 그래프"() -> (w391:refnum<vi>)
                n191 = property class="XYGraph (엄격한)"(reference=w391) -> ("CrsrList"=w392:T3)  [unwired: 1 in, 2 out]
                n192 = call "Buffer_Control.vi"("Mode"=buffer_mode."Output") -> ("Counts out"=w387:u32[][], "Timeline out"=w389:dbl[])  [unwired: 6 in, 3 out]
                n193 = Index Array(array=w392) -> (element #1=w393:T4, element #2=w394:T4)  [unwired: 2 in]
                n194 = Unbundle By Name(w393) -> ("Index"=w369:i32)
                n195 = Unbundle By Name(w394) -> ("Index"=w368:i32)
                n196 = Index Array(array=w387, index (row)=w386) -> (element=w385:u32[])  [unwired: 1 in]
                n197 = Subtract(x=w368, y=w369) -> (x-y=w382:i32)
                n198 = Index Array(array=w389, index #1=w369, index #2=w368) -> (element #1=w380:dbl, element #2=w379:dbl)
                n199 = Increment(x=w382) -> (x+1=w371:i32)
                n200 = Array Subset(array=w385, index=w369, length=w371) -> (w384:u32[])
                n201 = To Double Precision Float(number=w384) -> (double precision float=w383:dbl[])
                n202 = call-poly <vilib>:"Mean.vi"("X"=w383) -> ("mean"=w381:dbl)  [unwired: 1 out]
                n203 = Number To Fractional String(number=w381) -> (F-format string=w375:string)  [unwired: 3 in]
                n204 = Number To Fractional String(number=w380) -> (F-format string=w378:string)  [unwired: 3 in]
                n205 = Number To Fractional String(number=w379) -> (F-format string=w377:string)  [unwired: 3 in]
                n206 = Number To Decimal String(number=w371) -> (decimal integer string=w376:string)  [unwired: 1 in]
                n207 = Build Array(w378, w377, w376, w375) -> (w372:string[])
                n208 = Insert Into Array(array=w374, index (row)=w373, new element=w372) -> (w367:string[][])  [unwired: 1 in]
                n209 = call "Buffer_Index.vi"("Mode"=enum16{"Clear", "Add", "Del"}."Add", "End Index"=w368, "Start Index"=w369) -> ()  [unwired: 8 in, 1 out]
                n210 = call "SUB_SORT_2D_ARRAY.vi"("array"=w367) -> ("Sorted array"=w366:string[][])  [unwired: 10 in]
                n211 = property class="MCListbox (엄격한)"(reference=w388, "ItemNames"=w366) -> ()  [unwired: 1 in, 2 out]
              }
            }
          }
        }
        n212 = Enqueue Element(queue=w334, element="Idle", error in (no error)=w335) -> (error out=w336:errorcluster)  [unwired: 1 in, 2 out]
      }
      frame "Clear Table" {
        n213 = Two Button Dialog(message="Clear?" ("메시지")) -> (T button?=w395:bool)  [unwired: 2 in]
        n214 = case shown="거짓" w395 {
          frame False {
          }
          frame True {
            n215 = control-ref of="Analysis List"() -> (w402:refnum<vi>)
            n216 = property class="MCListbox (엄격한)"(reference=w402, "ItemNames"=string[][] []) -> ()  [unwired: 1 in, 2 out]
          }
        }
        n217 = Enqueue Element(queue=w397, element="Idle", error in (no error)=w398) -> (error out=w399:errorcluster)  [unwired: 1 in, 2 out]
      }
      frame "Auto Range Setting" {
        n218 = control-ref of="Plot Display mode"() -> (w404:refnum<vi>)
        n219 = property class="Enum (엄격한)"(reference=w404) -> ("Value"=w403:T1)  [unwired: 1 in, 2 out]
        n220 = case shown="\"Left A\", 기본" w403 {
          frame "All" {
            n221 = One Button Dialog(message="Plot Display mode must be not All~!" ("메시지")) -> ()  [unwired: 1 in, 1 out]
          }
          frame "Left A", Default {
            n222 = stacked-sequence {
              seq-local: [w413 _ _ _ _] -> [_ w442 _ _ _]
              seq-local: [_ w431 _ _ _] -> [_ _ w451 w499 _]
              seq-local: [_ w433 _ _ _] -> [_ _ w450 w498 _]
              seq-local: [_ w432 _ _ _] -> [_ _ w453 _ _]
              seq-local: [_ _ _ w495 _] -> [_ _ _ _ w522]
              seq-local: [w410 _ _ _ _] -> [_ _ w454 _ _]
              seq-local: [_ _ w452 _ _] -> [_ _ _ w494 _]
              seq-local: [_ w423 _ _ _] -> [_ _ w449 _ _]
              frame #0 {
                # "Search data will be used"
                n223 = property on="Analysis mode" class="Ring (엄격한)"() -> ("RingText.Text"=w410:string)  [unwired: 2 in, 2 out]
                n224 = control-ref of="Use Filter data"() -> (w415:refnum<vi>)
                n225 = control-ref of="Plot Display mode"() -> (w416:refnum<vi>)
                n226 = property class="Bool (엄격한)"(reference=w415) -> ("Value"=w414:bool)  [unwired: 1 in, 2 out]
                n227 = property class="Enum (엄격한)"(reference=w416) -> ("Value"=w412:T1)  [unwired: 1 in, 2 out]
                n228 = To Long Integer(number=w412) -> (32bit integer=w411:i32)
                n229 = case shown="참" w414 {
                  tunnel: w411 -> [w418 w419]
                  tunnel: [w417 w420] -> w413
                  frame False {
                    n230 = Decrement(x=w418) -> (x-1=w417:i32)
                  }
                  frame True {
                    # "If Left A, 6\n1 + 5 = 6"
                    n231 = Add(x=5, y=w419) -> (x+y=w420:i32)
                  }
                }
              }
              frame #1 {
                # "Min -> Sec -> ms"
                # "Check the Time Interval of Data -> Search Changing Point -> Apply Offset"
                n232 = call "Buffer_Control.vi"("Mode"=buffer_mode."Output") -> ("Counts out"=w437:u32[][], "Timeline out"=w431:dbl[])  [unwired: 6 in, 3 out]
                n233 = Index Array(array=w431, index #1=0 ("인덱스"), index #2=199 ("인덱스")) -> (element #1=w427:dbl, element #2=w428:dbl)
                n234 = Subtract(x=w428, y=w427) -> (x-y=w426:dbl)
                n235 = Divide(x=w426, y=200.0) -> (x/y=w424:dbl)
                n236 = Multiply(x=60.0, y=w424) -> (x*y=w439:dbl)
                n237 = Index Array(array=w437, index (row)=w442) -> (element=w433:u32[])  [unwired: 1 in]
                n238 = Multiply(x=w439, y=1000.0) -> (x*y=w423:dbl)
                n239 = call "Sub_Seach_Changing_Point.vi"("Data Interval Time(ms)"=w423, "Reverse Search?"=TRUE, "Input Array"=w433) -> ("Output"=w436:i32[])  [unwired: 8 in]
                n240 = disable-structure shown="활성화" {
                  disable-tunnel: [w444 0] -> w435
                  disable-tunnel: w431 -> [w443 _]
                  frame Disabled {
                    # "Offset of x AND Number of Data for 10 Sec"
                    # "Offset Time = 10Sec = 0.1667"
                    n241 = Threshold 1D Array(2:0.1667 ("임계점 y"), 3:w443) -> (0:w446:dbl)  [unwired: 1 in]
                    n242 = Round Toward +Infinity(x=w446) -> (ceil(x): smallest int >= x=w445:dbl)
                    n243 = To Long Integer(number=w445) -> (32bit integer=w444:i32)
                  }
                  frame Enabled {
                  }
                }
                n244 = Insert Into Array(array=w436, index=0 ("인덱스"), new element=w435) -> (w432:i32[])
              }
              frame #2 {
                n245 = case shown="\"Reated Loading\"" w454 {
                  tunnel: w453 -> [w455 w462]
                  tunnel: [w455 w459] -> w452
                  tunnel: w451 -> [_ w467]
                  tunnel: w450 -> [_ w466]
                  tunnel: w449 -> [_ w465]
                  frame "", Default {
                  }
                  frame "Reated Loading" {
                    # "Repeat 9 Times"
                    n246 = Delete From Array(array=w462, length=4 ("길이"), index=0 ("인덱스")) -> (deleted portion=w461:i32[])  [unwired: 1 out]
                    n247 = for {
                      N: 9 -> [_]
                      tunnel: w467 -> [w490]
                      tunnel: w466 -> [w485]
                      shift-right: [w476] -> w457
                      shift-left: w462 -> [w480]
                      tunnel: w465 -> [w483]
                      shift-right: [w479] -> w460
                      shift-left: w461 -> [w478]
                      tunnel: [w473] -> w458
                      stop <- w473 stop-if-true
                      # "Search 4 changing points"
                      # "Put removed data index value + chaning point into Shift reg 0"
                      # "Remove data From Orignal Data (previous End Time of 4th row data + 0.44min)"
                      n248 = Index Array(array=w480, index=3 ("인덱스")) -> (element=w474:i32)
                      n249 = Index Array(array=w490, index=w474) -> (element=w492:dbl)
                      n250 = Equal To 0?(x=w474) -> (x = 0?=w473:bool)
                      n251 = expression code="x+0.1667+0.6667+0.42"(w492) -> (w491:dbl)
                      n252 = Threshold 1D Array(2:w491, 3:w490) -> (0:w489:dbl)  [unwired: 1 in]
                      n253 = Add(x=w489, y=0.5) -> (x+y=w487:dbl)
                      n254 = Round Toward -Infinity(1:w487) -> (0:w486:dbl)
                      n255 = To Long Integer(number=w486) -> (32bit integer=w481:i32)
                      n256 = Delete From Array(array=w485, length=w481, index=0 ("인덱스")) -> (array with subset deleted=w482:u32[])  [unwired: 1 out]
                      n257 = call "Sub_Seach_Changing_Point.vi"("Data Interval Time(ms)"=w483, "Reverse Search?"=FALSE, "Input Array"=w482) -> ("Output"=w475:i32[])  [unwired: 8 in]
                      n258 = Add(x=w475, y=w481) -> (x+y=w476:i32[])
                      n259 = Build Array (concatenate)(w478, w476) -> (w479:i32[])
                    }
                    n260 = Array Size(array=w457) -> (size(s)=w456:i32)
                    n261 = case shown="참" w458 {
                      tunnel: w460 -> [w469 w472]
                      tunnel: [w469 w471] -> w459
                      tunnel: w456 -> [_ w470]
                      frame False {
                      }
                      frame True {
                        n262 = Delete From Array(array=w472, length=w470) -> (array with subset deleted=w471:i32[])  [unwired: 1 in, 1 out]
                      }
                    }
                  }
                }
              }
              frame #3 {
                # "Range"
                # "Time\nCounts"
                # "Table Data Calculation"
                n263 = Array Size(array=w494) -> (size(s)=w497:i32)
                n264 = Decrement(x=w497) -> (x-1=w496:i32)
                n265 = for {
                  N: w496 -> [_]
                  tunnel: w494 -> [w520] mode=indexing
                  tunnel: w499 -> [w514]
                  tunnel: w498 -> [w511]
                  tunnel: [w501] -> w495 mode=indexing
                  # "Average"
                  # "Number of Sample"
                  # "End Time"
                  # "10Sec = 0.1667min\n40Sec = 0.6667min"
                  # "Start Time"
                  n266 = Index Array(array=w514, index=w520) -> (element=w515:dbl)
                  n267 = Add(x=w515, y=0.1667 ("임계점 y")) -> (x+y=w500:dbl)
                  n268 = Add(x=w500, y=0.6667) -> (x+y=w504:dbl)
                  n269 = Threshold 1D Array(2:w500, 3:w514) -> (0:w519:dbl)  [unwired: 1 in]
                  n270 = Threshold 1D Array(2:w504, 3:w514) -> (0:w512:dbl)  [unwired: 1 in]
                  n271 = Round Toward +Infinity(x=w519) -> (ceil(x): smallest int >= x=w518:dbl)
                  n272 = Round Toward +Infinity(x=w512) -> (ceil(x): smallest int >= x=w513:dbl)
                  n273 = To Long Integer(number=w518) -> (32bit integer=w509:i32)
                  n274 = To Long Integer(number=w513) -> (32bit integer=w510:i32)
                  n275 = Subtract(x=w510, y=w509) -> (x-y=w508:i32)
                  n276 = Increment(x=w508) -> (x+1=w505:i32)
                  n277 = Array Subset(array=w511, index=w509, length=w505) -> (w507:u32[])
                  n278 = To Double Precision Float(number=w507) -> (double precision float=w506:dbl[])
                  n279 = To Double Precision Float(number=w505) -> (double precision float=w503:dbl)
                  n280 = call-poly <vilib>:"Mean.vi"("X"=w506) -> ("mean"=w502:dbl)  [unwired: 1 out]
                  n281 = Build Array(w500, w504, w503, w502) -> (w501:dbl[])
                }
              }
              frame #4 {
                # "Add List"
                n282 = for {
                  tunnel: w522 -> [w534] mode=indexing
                  tunnel: [w523] -> w521 mode=indexing
                  w530 = i16 4 ("정밀도(6)")
                  n283 = Index Array(array=w534) -> (element #1=w533:dbl, element #2=w532:dbl, element #3=w529:dbl, element #4=w531:dbl)  [unwired: 4 in]
                  n284 = To Long Integer(number=w529) -> (32bit integer=w528:i32)
                  n285 = Number To Fractional String(number=w533, precision (6)=w530) -> (F-format string=w527:string)  [unwired: 2 in]
                  n286 = Number To Fractional String(number=w532, precision (6)=w530) -> (F-format string=w526:string)  [unwired: 2 in]
                  n287 = Number To Fractional String(number=w531, precision (6)=w530) -> (F-format string=w524:string)  [unwired: 2 in]
                  n288 = Number To Decimal String(number=w528) -> (decimal integer string=w525:string)  [unwired: 1 in]
                  n289 = Build Array(w527, w526, w525, w524) -> (w523:string[])
                }
                n290 = property on="Analysis List" class="MCListbox (엄격한)"("ItemNames"=w521) -> ()  [unwired: 2 in, 2 out]
              }
            }
          }
        }
        n291 = Enqueue Element(queue=w405, element="Idle", error in (no error)=w406) -> (error out=w407:errorcluster)  [unwired: 1 in, 2 out]
      }
      frame "Move to Cursor" {
        n292 = control-ref of="Analysis List"() -> (w554:refnum<vi>)
        n293 = control-ref of="XY 그래프"() -> (w549:refnum<vi>)
        n294 = property class="XYGraph (엄격한)"(reference=w549) -> (reference out=w561:refnum<vi>, error out=w568:errorcluster, "CrsrList"=w562:T3)  [unwired: 1 in]
        n295 = property class="MCListbox (엄격한)"(reference=w554) -> ("FocusRow"=w556:i32)  [unwired: 1 in, 2 out]
        n296 = property on="Analysis List" class="MCListbox (엄격한)"() -> ("ItemNames"=w555:string[][])  [unwired: 2 in, 2 out]
        n297 = Index Array(array=w562) -> (element #1=w564:T4, element #2=w563:T4)  [unwired: 2 in]
        n298 = Index Array(array=w555, index (row) #1=w556, index (col) #1=0 ("비활성화된 인덱스 (열)"), index (row) #2=w556, index (col) #2=1 ("비활성화된 인덱스 (열)")) -> (element #1=w559:string, element #2=w560:string)
        n299 = Fract/Exp String To Number(string=w559) -> (number=w548:dbl)  [unwired: 3 in, 1 out]
        n300 = Fract/Exp String To Number(string=w560) -> (number=w546:dbl)  [unwired: 3 in, 1 out]
        n301 = call "Buffer_Control.vi"("Mode"=buffer_mode."Output") -> ("Timeline out"=w547:dbl[])  [unwired: 6 in, 4 out]
        n302 = Threshold 1D Array(2:w548, 3:w547) -> (0:w542:dbl)  [unwired: 1 in]
        n303 = Threshold 1D Array(2:w546, 3:w547) -> (0:w543:dbl)  [unwired: 1 in]
        n304 = Add(x=w542, y=0.5) -> (x+y=w540:dbl)
        n305 = Add(x=w543, y=0.5) -> (x+y=w541:dbl)
        n306 = Round Toward -Infinity(1:w540) -> (0:w539:dbl)
        n307 = Round Toward -Infinity(1:w541) -> (0:w538:dbl)
        n308 = To Long Integer(number=w538) -> (32bit integer=w536:i32)
        n309 = To Long Integer(number=w539) -> (32bit integer=w537:i32)
        n310 = Bundle By Name(cluster=w563, "Index"=w536) -> (w565:T4)
        n311 = Bundle By Name(cluster=w564, "Index"=w537) -> (w566:T4)
        n312 = Build Array(w566, w565) -> (w567:T9)
        n313 = property class="XYGraph (엄격한)"(reference=w561, error in=w568, "CrsrList"=w567) -> ()  [unwired: 2 out]
        n314 = Enqueue Element(queue=w550, element="Idle", error in (no error)=w551) -> (error out=w552:errorcluster)  [unwired: 1 in, 2 out]
      }
      frame "Analysis" {
        n315 = stacked-sequence {
          seq-local: [_ w575 _ _] -> [_ _ w595 _]
          frame #0 {
            n316 = call <vilib>:"Set Busy.vi"() -> ()  [unwired: 10 in, 2 out]
          }
          frame #1 {
            n317 = property on="Analysis mode" class="Ring (엄격한)"() -> ("RingText.Text"=w574:string)  [unwired: 2 in, 2 out]
            n318 = case shown="\"Variation with Changing Voltage\"" w574 {
              tunnel: ["" ("이름 또는 상대 경로") "Sensor Response Linearity.xlsx" ("이름 또는 상대 경로") "Sensor Hysteresis.xlsx" ("이름 또는 상대 경로") "Reated Loading.xlsx" ("이름 또는 상대 경로") "Electrical Noise.xlsx" ("이름 또는 상대 경로") "Variation Due to Self-Heating.xlsx" ("이름 또는 상대 경로") "Variation with Changing Voltage.xlsx" ("이름 또는 상대 경로") "Drift with Set Temperature and Voltage.xlsx" ("이름 또는 상대 경로")] -> w576
              tunnel: [0 ("row") 28 ("row") 28 ("row") 78 ("row") 28 ("row") 35 ("row") 53 ("row") 28 ("row")] -> w573
              frame "", Default {
              }
              frame "Sensor Response Linearity" {
              }
              frame "Sensor Hysteresis with No Dwell Time", "Sensor Hysteresis with Varying Dwell Time" {
              }
              frame "Reated Loading" {
              }
              frame "Electrical Noise" {
              }
              frame "Variation Due to Self-Heating" {
              }
              frame "Variation with Changing Voltage" {
              }
              frame "Drift with Set Temperature and Voltage" {
              }
            }
            n319 = control-ref of="File Name"() -> (w577:refnum<vi>)
            n320 = control-ref of="File Path"() -> (w578:refnum<vi>)
            n321 = call "Sub_Saveas.vi"("Template Name"=w576, "row"=w573, "File Name"=w577, "Path"=w578) -> ("Save Path"=w575:path)  [unwired: 7 in]
          }
          frame #2 {
            n322 = property on="Analysis mode" class="Ring (엄격한)"() -> ("RingText.Text"=w598:string)  [unwired: 2 in, 2 out]
            n323 = control-ref of="Use Filter data"() -> (w597:refnum<vi>)
            n324 = property class="Bool (엄격한)"(reference=w597) -> ("Value"=w596:bool)  [unwired: 1 in, 2 out]
            n325 = case shown="\"Variation with Changing Voltage\"" w598 {
              tunnel: w596 -> [_ w611 w651 w680 w748 w792 w816 w838]
              tunnel: w595 -> [_ w603 w643 w679 w747 w783 w805 w837]
              frame "", Default {
              }
              frame "Sensor Response Linearity" {
                n326 = property on="Analysis List" class="MCListbox (엄격한)"() -> ("ItemNames"=w612:string[][])  [unwired: 2 in, 2 out]
                n327 = case shown="거짓" w611 {
                  tunnel: [36 43] -> w606
                  frame False {
                  }
                  frame True {
                  }
                }
                n328 = control-ref of="Plot Display mode"() -> (w610:refnum<vi>)
                n329 = property class="Enum (엄격한)"(reference=w610) -> ("Value"=w609:T1)  [unwired: 1 in, 2 out]
                n330 = To Long Integer(number=w609) -> (32bit integer=w608:i32)
                n331 = Decrement(x=w608) -> (x-1=w607:i32)
                n332 = Add(x=w607, y=w606) -> (x+y=w605:i32)
                n333 = call "col number conversion.vi"("Col Number"=w605) -> ("Excel Col Number"=w604:string)  [unwired: 10 in]
                n334 = for {
                  tunnel: w612 -> [w638] mode=indexing
                  tunnel: w604 -> [w618]
                  tunnel: [w615] -> w602 mode=indexing
                  # "Offset"
                  n335 = Index Array(array=w638) -> (element #1=w636:string, element #2=w637:string)  [unwired: 2 in]
                  n336 = call "Buffer_Control.vi"("Mode"=buffer_mode."Output") -> ("Timeline out"=w632:dbl[])  [unwired: 6 in, 4 out]
                  n337 = Fract/Exp String To Number(string=w636) -> (number=w635:dbl)  [unwired: 3 in, 1 out]
                  n338 = Fract/Exp String To Number(string=w637) -> (number=w634:dbl)  [unwired: 3 in, 1 out]
                  n339 = Threshold 1D Array(2:w635, 3:w632) -> (0:w629:dbl)  [unwired: 1 in]
                  n340 = Threshold 1D Array(2:w634, 3:w632) -> (0:w624:dbl)  [unwired: 1 in]
                  n341 = Add(x=w629, y=0.5) -> (x+y=w631:dbl)
                  n342 = Add(x=w624, y=0.5) -> (x+y=w625:dbl)
                  n343 = Round Toward -Infinity(1:w631) -> (0:w630:dbl)
                  n344 = Round Toward -Infinity(1:w625) -> (0:w626:dbl)
                  n345 = To Long Integer(number=w630) -> (32bit integer=w623:i32)
                  n346 = To Long Integer(number=w626) -> (32bit integer=w621:i32)
                  n347 = Add(x=w623, y=29) -> (x+y=w617:i32)
                  n348 = Add(x=w621, y=29) -> (x+y=w616:i32)
                  n349 = Format Into String(format string="=AVERAGE(%s$%d:%s$%d)" ("포맷 문자열"), w618, w617, w618, w616) -> (resulting string=w615:string)  [unwired: 2 in, 1 out]
                }
                n350 = Build Array(w602) -> (w601:string[][])
                n351 = Transpose 2D Array(2D array=w601) -> (transposed array=w600:string[][])
                n352 = call "Save_Text_Array_to_Excel.vi"("MS Office parameters"=T6 {"position (excel)"={"row"=3, "column"=2}, "name (excel)"="", "bookmark (word)"=""}, "Array"=w600, "Save Path"=w603) -> ()  [unwired: 9 in]
              }
              frame "Sensor Hysteresis with No Dwell Time", "Sensor Hysteresis with Varying Dwell Time" {
                n353 = property on="Analysis List" class="MCListbox (엄격한)"() -> ("ItemNames"=w652:string[][])  [unwired: 2 in, 2 out]
                n354 = case shown="거짓" w651 {
                  tunnel: [36 43] -> w646
                  frame False {
                  }
                  frame True {
                  }
                }
                n355 = control-ref of="Plot Display mode"() -> (w650:refnum<vi>)
                n356 = property class="Enum (엄격한)"(reference=w650) -> ("Value"=w649:T1)  [unwired: 1 in, 2 out]
                n357 = To Long Integer(number=w649) -> (32bit integer=w648:i32)
                n358 = Decrement(x=w648) -> (x-1=w647:i32)
                n359 = Add(x=w647, y=w646) -> (x+y=w645:i32)
                n360 = call "col number conversion.vi"("Col Number"=w645) -> ("Excel Col Number"=w644:string)  [unwired: 10 in]
                n361 = for {
                  tunnel: w652 -> [w678] mode=indexing
                  tunnel: w644 -> [w658]
                  tunnel: [w655] -> w642 mode=indexing
                  # "Offset"
                  n362 = Index Array(array=w678) -> (element #1=w676:string, element #2=w677:string)  [unwired: 2 in]
                  n363 = call "Buffer_Control.vi"("Mode"=buffer_mode."Output") -> ("Timeline out"=w672:dbl[])  [unwired: 6 in, 4 out]
                  n364 = Fract/Exp String To Number(string=w676) -> (number=w675:dbl)  [unwired: 3 in, 1 out]
                  n365 = Fract/Exp String To Number(string=w677) -> (number=w674:dbl)  [unwired: 3 in, 1 out]
                  n366 = Threshold 1D Array(2:w675, 3:w672) -> (0:w669:dbl)  [unwired: 1 in]
                  n367 = Threshold 1D Array(2:w674, 3:w672) -> (0:w664:dbl)  [unwired: 1 in]
                  n368 = Add(x=w669, y=0.5) -> (x+y=w671:dbl)
                  n369 = Add(x=w664, y=0.5) -> (x+y=w665:dbl)
                  n370 = Round Toward -Infinity(1:w671) -> (0:w670:dbl)
                  n371 = Round Toward -Infinity(1:w665) -> (0:w666:dbl)
                  n372 = To Long Integer(number=w670) -> (32bit integer=w663:i32)
                  n373 = To Long Integer(number=w666) -> (32bit integer=w661:i32)
                  n374 = Add(x=w663, y=29) -> (x+y=w657:i32)
                  n375 = Add(x=w661, y=29) -> (x+y=w656:i32)
                  n376 = Format Into String(format string="=AVERAGE(%s$%d:%s$%d)" ("포맷 문자열"), w658, w657, w658, w656) -> (resulting string=w655:string)  [unwired: 2 in, 1 out]
                }
                n377 = Build Array(w642) -> (w641:string[][])
                n378 = Transpose 2D Array(2D array=w641) -> (transposed array=w640:string[][])
                n379 = call "Save_Text_Array_to_Excel.vi"("MS Office parameters"=T6 {"position (excel)"={"row"=2, "column"=3}, "name (excel)"="", "bookmark (word)"=""}, "Array"=w640, "Save Path"=w643) -> ()  [unwired: 9 in]
              }
              frame "Reated Loading" {
                n380 = stacked-sequence {
                  seq-local: [w681 _] -> [_ w730]
                  tunnel: w680 -> [w689 _]
                  tunnel: w679 -> [_ w717]
                  frame #0 {
                    n381 = property on="Analysis List" class="MCListbox (엄격한)"() -> ("ItemNames"=w690:string[][])  [unwired: 2 in, 2 out]
                    n382 = case shown="거짓" w689 {
                      tunnel: [36 43] -> w684
                      frame False {
                      }
                      frame True {
                      }
                    }
                    n383 = control-ref of="Plot Display mode"() -> (w688:refnum<vi>)
                    n384 = property class="Enum (엄격한)"(reference=w688) -> ("Value"=w687:T1)  [unwired: 1 in, 2 out]
                    n385 = To Long Integer(number=w687) -> (32bit integer=w686:i32)
                    n386 = Decrement(x=w686) -> (x-1=w685:i32)
                    n387 = Add(x=w685, y=w684) -> (x+y=w683:i32)
                    n388 = call "col number conversion.vi"("Col Number"=w683) -> ("Excel Col Number"=w682:string)  [unwired: 10 in]
                    n389 = for {
                      tunnel: w690 -> [w716] mode=indexing
                      tunnel: w682 -> [w696]
                      tunnel: [w693] -> w681 mode=indexing
                      # "Offset"
                      n390 = Index Array(array=w716) -> (element #1=w714:string, element #2=w715:string)  [unwired: 2 in]
                      n391 = call "Buffer_Control.vi"("Mode"=buffer_mode."Output") -> ("Timeline out"=w710:dbl[])  [unwired: 6 in, 4 out]
                      n392 = Fract/Exp String To Number(string=w714) -> (number=w713:dbl)  [unwired: 3 in, 1 out]
                      n393 = Fract/Exp String To Number(string=w715) -> (number=w712:dbl)  [unwired: 3 in, 1 out]
                      n394 = Threshold 1D Array(2:w713, 3:w710) -> (0:w707:dbl)  [unwired: 1 in]
                      n395 = Threshold 1D Array(2:w712, 3:w710) -> (0:w702:dbl)  [unwired: 1 in]
                      n396 = Add(x=w707, y=0.5) -> (x+y=w709:dbl)
                      n397 = Add(x=w702, y=0.5) -> (x+y=w703:dbl)
                      n398 = Round Toward -Infinity(1:w709) -> (0:w708:dbl)
                      n399 = Round Toward -Infinity(1:w703) -> (0:w704:dbl)
                      n400 = To Long Integer(number=w708) -> (32bit integer=w701:i32)
                      n401 = To Long Integer(number=w704) -> (32bit integer=w699:i32)
                      n402 = Add(x=w701, y=29) -> (x+y=w695:i32)
                      n403 = Add(x=w699, y=29) -> (x+y=w694:i32)
                      n404 = Format Into String(format string="=AVERAGE(%s$%d:%s$%d)" ("포맷 문자열"), w696, w695, w696, w694) -> (resulting string=w693:string)  [unwired: 2 in, 1 out]
                    }
                  }
                  frame #1 {
                    n405 = Reshape Array(w730, 10 ("차원 크기"), 4 ("차원 크기")) -> (w729:string[][])
                    n406 = Transpose 2D Array(2D array=w729) -> (transposed array=w728:string[][])
                    n407 = call <vilib>:"New Report.vi"("window state (normal)"=T7."no change", "report type"=T8."Excel", "template (empty)"=w717) -> ("report out"=w723:refnum<class "NI_report.lvclass">, "error out"=w724:errorcluster)  [unwired: 11 in]
                    n408 = for {
                      tunnel: w728 -> [w745] mode=indexing
                      tunnel: 6 -> [w740]
                      shift-right: [w736] -> w718
                      shift-left: w723 -> [w735]
                      shift-right: [w733] -> w719
                      shift-left: w724 -> [w734]
                      i -> [w742]
                      n409 = Multiply(x=w742, y=17) -> (x*y=w741:i32)
                      n410 = Add(x=w740, y=w741) -> (x+y=w739:i32)
                      n411 = Bundle By Name(cluster=T6 {"position (excel)"={"row"=2, "column"=3}, "name (excel)"="", "bookmark (word)"=""} ("MS Office parameters"), "position (excel).row"=w739) -> (w737:T6)
                      n412 = Build Array(w745) -> (w746:string[][])
                      n413 = Transpose 2D Array(2D array=w746) -> (transposed array=w738:string[][])
                      n414 = call-poly <vilib>:"Append Table to Report.vi"("report in"=w735, "MS Office parameters"=w737, "text data"=w738, "error in (no error)"=w734) -> ("report out"=w736:refnum<class "NI_report.lvclass">, "error out"=w733:errorcluster)  [unwired: 8 in, 2 out]
                    }
                    n415 = call-dynamic "Save Report to File.vi"("report in"=w718, "report file path"=w717, "prompt to replace? (F)"=FALSE, "error in (no error)"=w719) -> ("report out"=w721:refnum<class "NI_report.lvclass">, "error out"=w720:errorcluster)  [unwired: 10 in]
                    n416 = call-dynamic "Dispose Report.vi"("report in"=w721, "error in (no error)"=w720) -> ()  [unwired: 13 in, 1 out]
                  }
                }
              }
              frame "Electrical Noise" {
                n417 = stacked-sequence {
                  seq-local: [w749 _] -> [_ w776]
                  tunnel: w748 -> [w751 _]
                  tunnel: w747 -> [_ w777]
                  frame #0 {
                    # "Time for analysis"
                    n418 = for {
                      tunnel: i32[] [0, 10, 20, 30] -> [w762] mode=indexing
                      tunnel: w751 -> [w763]
                      shift-right: [w759] -> w749
                      shift-left: string[][] [] -> [w758]
                      i -> [w755]
                      # "Col"
                      # "Start Point\nRow = 29"
                      n419 = case shown="참" w763 {
                        tunnel: [36 43] -> w760
                        frame False {
                        }
                        frame True {
                        }
                      }
                      n420 = case shown="1.., 기본" w762 {
                        selector: w762 -> [_ w772]
                        tunnel: [38 w765] -> w761
                        frame 0 {
                        }
                        frame 1.., Default {
                          n421 = call "Buffer_Control.vi"("Mode"=buffer_mode."Output") -> ("Timeline out"=w770:dbl[])  [unwired: 6 in, 4 out]
                          n422 = To Double Precision Float(number=w772) -> (double precision float=w771:dbl)
                          n423 = Subtract(x=w770, y=w771) -> (x-y=w769:dbl[])
                          n424 = Absolute Value(x=w769) -> (abs(x)=w768:dbl[])
                          n425 = Array Max & Min(array=w768) -> (min index (indices)=w767:i32)  [unwired: 3 out]
                          n426 = Add(x=29, y=w767) -> (x+y=w765:i32)
                        }
                      }
                      n427 = call "Sub_Electrical_Noise_Analysis-Excel-1.vi"("Init Col Value"=w760, "Init Row Value"=w761) -> ("Output"=w757:string[][])  [unwired: 9 in]
                      n428 = call "Sub_Electrical_Noise_Analysis-Excel-2.vi"("iteration(0)"=w755) -> ("Output"=w756:string[])  [unwired: 10 in]
                      n429 = Insert Into Array(array=w757, index (row)=3 ("인덱스 (행)"), new element=w756) -> (w754:string[][])  [unwired: 1 in]
                      n430 = Build Array (concatenate)(w758, w754) -> (w759:string[][])
                    }
                  }
                  frame #1 {
                    n431 = call "Save_Text_Array_to_Excel.vi"("MS Office parameters"=T6 {"position (excel)"={"row"=2, "column"=2}, "name (excel)"="", "bookmark (word)"=""}, "Array"=w776, "Save Path"=w777) -> ()  [unwired: 9 in]
                  }
                }
              }
              frame "Drift with Set Temperature and Voltage" {
                w784 = 29 ("y")
                # "Last Data Position + offset(29)"
                # "Row"
                # "Col"
                n432 = case shown="거짓" w792 {
                  tunnel: [36 43] -> w790
                  frame False {
                  }
                  frame True {
                  }
                }
                n433 = call "Buffer_Control.vi"("Mode"=buffer_mode."Output") -> ("Timeline out"=w788:dbl[])  [unwired: 6 in, 4 out]
                n434 = Array Size(array=w788) -> (size(s)=w787:i32)
                n435 = Decrement(x=w787) -> (x-1=w786:i32)
                n436 = Add(x=w784, y=w786) -> (x+y=w785:i32)
                n437 = call "col number conversion.vi"("Col Number"=35) -> ("Excel Col Number"=w780:string)  [unwired: 10 in]
                n438 = for {
                  N: 6 -> [_]
                  tunnel: w790 -> [w802]
                  tunnel: w785 -> [w793]
                  tunnel: w784 -> [w794]
                  tunnel: [w796] -> w779 mode=indexing
                  tunnel: w780 -> [w795]
                  i -> [w798]
                  n439 = Add(x=w802, y=w798) -> (x+y=w800:i32)
                  n440 = call "col number conversion.vi"("Col Number"=w800) -> ("Excel Col Number"=w799:string)  [unwired: 10 in]
                  n441 = Format Into String(format string="=SLOPE(%s$%d:%s$%d,%s$%d:%s$%d)/(24*60)" ("포맷 문자열"), w799, w794, w799, w793, w795, w794, w795, w793) -> (resulting string=w797:string)  [unwired: 2 in, 1 out]
                  n442 = Build Array(w797) -> (w796:string[])
                }
                n443 = call "Save_Text_Array_to_Excel.vi"("MS Office parameters"=T6 {"position (excel)"={"row"=4, "column"=1}, "name (excel)"="", "bookmark (word)"=""}, "Array"=w779, "Save Path"=w783) -> ()  [unwired: 9 in]
              }
              frame "Variation Due to Self-Heating" {
                w809 = 46 ("y")
                # "Last Data Position + offset(46)"
                # "Row"
                # "=INDEX(LINEST('Calculated Data'!$D10:$D571,'Calculated Data'!$C$10:$C$571^{1,2,3}),1,Position)\nPosition = 1~4"
                n444 = call "Buffer_Control.vi"("Mode"=buffer_mode."Output") -> ("Timeline out"=w812:dbl[])  [unwired: 6 in, 4 out]
                n445 = Array Size(array=w812) -> (size(s)=w811:i32)
                n446 = Decrement(x=w811) -> (x-1=w810:i32)
                n447 = Add(x=w809, y=w810) -> (x+y=w808:i32)
                n448 = case shown="거짓" w816 {
                  tunnel: [36 43] -> w814
                  frame False {
                  }
                  frame True {
                  }
                }
                n449 = for {
                  N: 4 -> [_]
                  tunnel: w814 -> [w822]
                  tunnel: w809 -> [w821]
                  tunnel: w808 -> [w820]
                  tunnel: [w817] -> w806 mode=indexing
                  i -> [w819]
                  n450 = Increment(x=w819) -> (x+1=w818:i32)
                  n451 = for {
                    N: 6 -> [_]
                    tunnel: w822 -> [w828]
                    tunnel: w821 -> [w830]
                    tunnel: w820 -> [w829]
                    tunnel: w818 -> [w825]
                    tunnel: [w824] -> w817 mode=indexing
                    i -> [w833]
                    n452 = Decrement(x=w828) -> (x-1=w827:i32)
                    n453 = Add(x=w828, y=w833) -> (x+y=w832:i32)
                    n454 = call "col number conversion.vi"("Col Number"=w827) -> ("Excel Col Number"=w826:string)  [unwired: 10 in]
                    n455 = call "col number conversion.vi"("Col Number"=w832) -> ("Excel Col Number"=w831:string)  [unwired: 10 in]
                    n456 = Format Into String(format string="=INDEX(LINEST(%s$%d:%s$%d,%s$%d:%s$%d^{1,2,3}),1,%d)" ("포맷 문자열"), w831, w830, w831, w829, w826, w830, w826, w829, w825) -> (resulting string=w824:string)  [unwired: 2 in, 1 out]
                  }
                }
                n457 = call "Save_Text_Array_to_Excel.vi"("MS Office parameters"=T6 {"position (excel)"={"row"=6, "column"=3}, "name (excel)"="", "bookmark (word)"=""}, "Array"=w806, "Save Path"=w805) -> ()  [unwired: 9 in]
              }
              frame "Variation with Changing Voltage" {
                n458 = stacked-sequence {
                  seq-local: [w839 _] -> [_ w876]
                  tunnel: w838 -> [w841 _]
                  tunnel: w837 -> [_ w875]
                  frame #0 {
                    # "Number of \nSensor = 6"
                    n459 = for {
                      N: 6 -> [_]
                      tunnel: [w847] -> w839 mode=indexing
                      tunnel: w841 -> [w844]
                      i -> [w845]
                      n460 = case shown="거짓" w844 {
                        tunnel: [36 43] -> w846
                        frame False {
                        }
                        frame True {
                        }
                      }
                      n461 = property on="Analysis List" class="MCListbox (엄격한)"() -> ("ItemNames"=w848:string[][])  [unwired: 2 in, 2 out]
                      n462 = Add(x=w845, y=w846) -> (x+y=w843:i32)
                      n463 = call "col number conversion.vi"("Col Number"=w843) -> ("Excel Col Number"=w842:string)  [unwired: 10 in]
                      n464 = for {
                        tunnel: w848 -> [w874] mode=indexing
                        tunnel: w842 -> [w854]
                        tunnel: [w851] -> w847 mode=indexing
                        # "Offset"
                        n465 = Index Array(array=w874) -> (element #1=w872:string, element #2=w873:string)  [unwired: 2 in]
                        n466 = call "Buffer_Control.vi"("Mode"=buffer_mode."Output") -> ("Timeline out"=w868:dbl[])  [unwired: 6 in, 4 out]
                        n467 = Fract/Exp String To Number(string=w872) -> (number=w871:dbl)  [unwired: 3 in, 1 out]
                        n468 = Fract/Exp String To Number(string=w873) -> (number=w870:dbl)  [unwired: 3 in, 1 out]
                        n469 = Threshold 1D Array(2:w871, 3:w868) -> (0:w865:dbl)  [unwired: 1 in]
                        n470 = Threshold 1D Array(2:w870, 3:w868) -> (0:w860:dbl)  [unwired: 1 in]
                        n471 = Add(x=w865, y=0.5) -> (x+y=w867:dbl)
                        n472 = Add(x=w860, y=0.5) -> (x+y=w861:dbl)
                        n473 = Round Toward -Infinity(1:w867) -> (0:w866:dbl)
                        n474 = Round Toward -Infinity(1:w861) -> (0:w862:dbl)
                        n475 = To Long Integer(number=w866) -> (32bit integer=w859:i32)
                        n476 = To Long Integer(number=w862) -> (32bit integer=w857:i32)
                        n477 = Add(x=w859, y=64) -> (x+y=w853:i32)
                        n478 = Add(x=w857, y=64) -> (x+y=w852:i32)
                        n479 = Format Into String(format string="=AVERAGE(%s$%d:%s$%d)" ("포맷 문자열"), w854, w853, w854, w852) -> (resulting string=w851:string)  [unwired: 2 in, 1 out]
                      }
                    }
                  }
                  frame #1 {
                    n480 = call <vilib>:"New Report.vi"("window state (normal)"=T7."no change", "report type"=T8."Excel", "template (empty)"=w875) -> ("report out"=w882:refnum<class "NI_report.lvclass">, "error out"=w883:errorcluster)  [unwired: 11 in]
                    n481 = for {
                      tunnel: w876 -> [w900] mode=indexing
                      tunnel: 1 -> [w895]
                      shift-right: [w891] -> w877
                      shift-left: w882 -> [w890]
                      shift-right: [w888] -> w878
                      shift-left: w883 -> [w889]
                      i -> [w897]
                      n482 = Multiply(x=w897, y=8) -> (x*y=w896:i32)
                      n483 = Add(x=w895, y=w896) -> (x+y=w894:i32)
                      n484 = Bundle By Name(cluster=T6 {"position (excel)"={"row"=2, "column"=3}, "name (excel)"="", "bookmark (word)"=""} ("MS Office parameters"), "position (excel).row"=w894, "position (excel).column"=2) -> (w892:T6)
                      n485 = Build Array(w900) -> (w901:string[][])
                      n486 = Transpose 2D Array(2D array=w901) -> (transposed array=w893:string[][])
                      n487 = call-poly <vilib>:"Append Table to Report.vi"("report in"=w890, "MS Office parameters"=w892, "text data"=w893, "error in (no error)"=w889) -> ("report out"=w891:refnum<class "NI_report.lvclass">, "error out"=w888:errorcluster)  [unwired: 8 in, 2 out]
                    }
                    n488 = call-dynamic "Save Report to File.vi"("report in"=w877, "report file path"=w875, "prompt to replace? (F)"=FALSE, "error in (no error)"=w878) -> ("report out"=w880:refnum<class "NI_report.lvclass">, "error out"=w879:errorcluster)  [unwired: 10 in]
                    n489 = call-dynamic "Dispose Report.vi"("report in"=w880, "error in (no error)"=w879) -> ()  [unwired: 13 in, 1 out]
                  }
                }
              }
            }
          }
          frame #3 {
            n490 = call <vilib>:"Unset Busy.vi"() -> ()  [unwired: 11 in, 1 out]
            n491 = One Button Dialog(message="Done~!!" ("메시지")) -> ()  [unwired: 1 in, 1 out]
          }
        }
        n492 = Enqueue Element(queue=w569, element="Idle", error in (no error)=w570) -> (error out=w571:errorcluster)  [unwired: 1 in, 2 out]
      }
    }
  }
  n493 = Flush Queue(queue=w4, error in (no error)=w3) -> (queue out=w6:refnum<queue>, error out=w5:errorcluster)  [unwired: 1 out]
  n494 = Release Queue(queue=w6, error in (no error)=w5) -> ()  [unwired: 1 in, 3 out]
